vi "900x 9870 Interrupt Read (Sub).vi"(8 "error in":errorcluster, 9 "Number of bytes":i32, 11 "FPGA In":T1) -> (0 "error out":errorcluster, 1 "Byte Count":u32, 2 "Read Bytes":string, 3 "FPGA Out":T1, 4 "Timed Out":bool, 6 "FPGA Error":errorcluster)   [LabVIEW 2012]
uses:
  900x INT FPGA Reference.ctl
  FPGA Function.ctl
  <vilib>/Utility/error.llb/Error Cluster From Error Code.vi
  <vilib>/rvi/errors/niLvFpgaAdjustHostInterfaceError.vi
  <vilib>/rvi/interface/nirviReadWriteControl/nirviReadWriteControl.xnode
  FPGA Bitfiles/NI-987xSerialLoo_FPGATarget3_9870InterfaceInt_BB93BC1A.lvbitx
  Program Files (x86)/National Instruments/LabVIEW 2012/examples/CompactRIO/Module Specific/NI 987x/Serial Loopback/VIs/9870 Interface Interrupt (FPGA).vi
  <vilib>/rvi/interface/nirviMethod/nirviMethod.xnode
  NiFpgaLv.dll
  <vilib>/FPGAPlugInAG/cRIO-9101/niLvFpga_AcknowledgeIrq_cRIO-9101.vi
  <vilib>/rvi/interface/nirviMethod/StockFPGA_InlinedMethodWaitForSingleIRQ.vi
  <vilib>/FPGAPlugInAG/cRIO-9101/niLvFpga_WaitOnIrq_cRIO-9101.vi
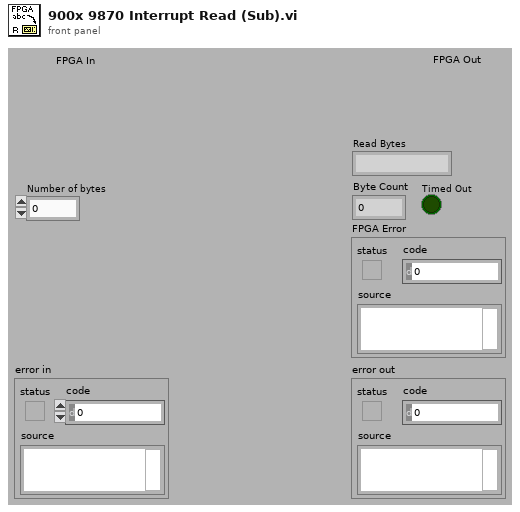
[diagram p1: front panel]
types:
  T1 = typedef "900x INT FPGA Reference.ctl" = refnum<k20>
  T2 = typedef "FPGA Function.ctl" = enum16{"Do Nothing", "Write", "Read"}
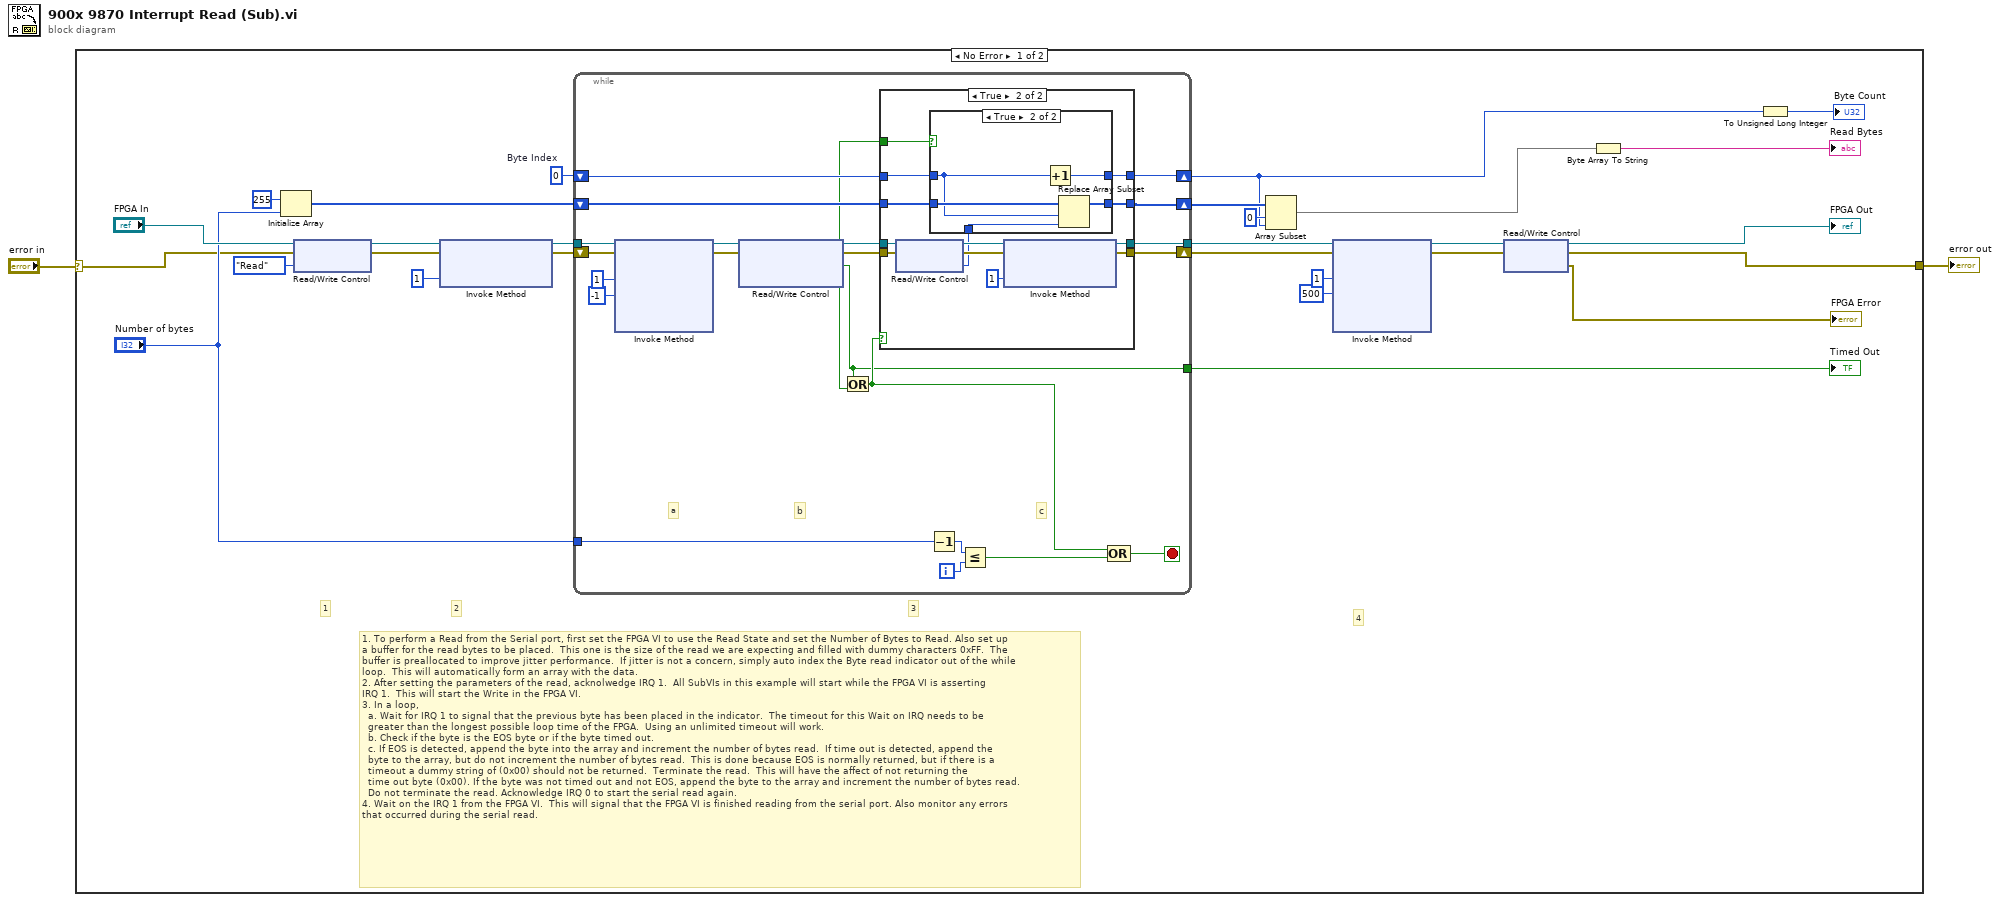
[diagram p0: block diagram]
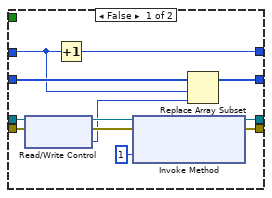
[diagram p2: hidden frame]
diagram:
  n1 = case shown="No Error" "error in" {
    selector: "error in" -> [w5 w85]
    tunnel: [w7 w85] -> w2
    frame No Error {
      w21 = 0  # Byte Index
      # "4"
      # "3"
      # "2"
      # "1"
      # "1. To perform a Read from the Serial port, first set the FPGA VI to use the Read State and set the Number of Bytes to Read. Also set up\na buffer for the read bytes to be placed.  This one is the size of the read we are expecting and filled with dummy characters 0xFF.  The\nbuffer is preallocated to improve jitter performance.  If jitter is not a concern, simply auto index the Byte read indicator out of the while\nloop.  This will automatically form an array with the data.\n2. After setting the parameters of the read, acknolwedge IRQ 1.  All SubVIs in this example will start while the FPGA VI is asserting \nIRQ 1.  This will start the Write in the FPGA VI.\n3. In a loop, \n  a. Wait for IRQ 1 to signal that the previous byte has been placed in the indicator.  The timeout for this Wait on IRQ needs to be\n  greater than the longest possible loop time of the FPGA.  Using an unlimited timeout will work.\n  b. Check if the byte is the EOS byte or if the byte timed out.\n  c. If EOS is detected, append the byte into the array and increment the number of bytes read.  If time out is detected, append the\n  byte to the array, but do not increment the number of bytes read.  This is done because EOS is normally returned, but if there is a \n  timeout a dummy string of (0x00) should not be returned.  Terminate the read.  This will have the affect of not returning the \n  time out byte (0x00). If the byte was not timed out and not EOS, append the byte to the array and increment the number of bytes read.  \n  Do not terminate the read. Acknowledge IRQ 0 to start the serial read again.\n4. Wait on the IRQ 1 from the FPGA VI.  This will signal that the FPGA VI is finished reading from the serial port. Also monitor any errors\nthat occurred during the serial read."
      n2 = Initialize Array(u8 255 ("element"), "Number of bytes") -> (w15:u8[])
      n3 = xnode "Read/Write Control"("FPGA VI Reference In"="FPGA In", "error in"=w5, "Op Control"=FPGA_Function."Read") -> ("FPGA VI Reference Out"=w29:T1, "error out"=w23:errorcluster)
      n4 = xnode "Invoke Method"("FPGA VI Reference In"=w29, "error in"=w23, "IRQ Number(s)"=1) -> ("FPGA VI Reference Out"=w28:T1, "error out"=w27:errorcluster)
      n5 = while {
        tunnel: [w52] -> w22
        shift-right: [w51] -> w24
        shift-left: w27 -> [w50]
        tunnel: w28 -> [w48]
        shift-right: [w46] -> w3
        shift-left: w21 -> [w47]
        tunnel: "Number of bytes" -> [w39]
        tunnel: [w32] -> w11
        shift-right: [w35] -> w14
        shift-left: w15 -> [w36]
        i -> [w40]
        stop <- w37 stop-if-true
        # "c"
        # "b"
        # "a"
        n6 = xnode "Invoke Method"("FPGA VI Reference In"=w48, "error in"=w50, "IRQ Number(s)"=1, "Timeout (ms)"=-1) -> ("FPGA VI Reference Out"=w45:T1, "error out"=w42:errorcluster)  [unwired: 2 out]
        n7 = xnode "Read/Write Control"("FPGA VI Reference In"=w45, "error in"=w42) -> ("FPGA VI Reference Out"=w44:T1, "error out"=w43:errorcluster, "Timed Out Read"=w32:bool, "EOS?"=w34:bool)
        n8 = Or(x=w32, y=w34) -> (x .or. y?=w33:bool)
        n9 = case shown="True" w33 {
          tunnel: [w64 w77] -> w52
          tunnel: [w63 w76] -> w51
          tunnel: w44 -> [w59 w72]
          tunnel: w43 -> [w58 w71]
          tunnel: w47 -> [w53 w66]
          tunnel: [w57 w67] -> w46
          tunnel: w36 -> [w55 w69]
          tunnel: [w56 w70] -> w35
          tunnel: w34 -> [_ w65]
          frame False {
            n10 = xnode "Read/Write Control"("FPGA VI Reference In"=w59, "error in"=w58) -> ("FPGA VI Reference Out"=w60:T1, "error out"=w61:errorcluster, "Byte read"=w54:u8)
            n11 = Increment(x=w53) -> (x+1=w57:i32)
            n12 = xnode "Invoke Method"("FPGA VI Reference In"=w60, "error in"=w61, "IRQ Number(s)"=1) -> ("FPGA VI Reference Out"=w64:T1, "error out"=w63:errorcluster)
            n13 = Replace Array Subset(array=w55, new element=w54, index=w53) -> (w56:u8[])
          }
          frame True {
            n14 = xnode "Read/Write Control"("FPGA VI Reference In"=w72, "error in"=w71) -> ("FPGA VI Reference Out"=w73:T1, "error out"=w74:errorcluster, "Byte read"=w68:u8)
            n15 = case shown="True" w65 {
              tunnel: [w79 w84] -> w70
              tunnel: w69 -> [w79 w83]
              tunnel: w68 -> [_ w82]
              tunnel: [w78 w80] -> w67
              tunnel: w66 -> [w78 w81]
              frame False {
              }
              frame True {
                n16 = Increment(x=w81) -> (x+1=w80:i32)
                n17 = Replace Array Subset(array=w83, new element=w82, index=w81) -> (w84:u8[])
              }
            }
            n18 = xnode "Invoke Method"("FPGA VI Reference In"=w73, "error in"=w74, "IRQ Number(s)"=1) -> ("FPGA VI Reference Out"=w77:T1, "error out"=w76:errorcluster)
          }
        }
        n19 = Decrement(x=w39) -> (x-1=w38:i32)
        n20 = Less Or Equal?(x=w38, y=w40) -> (x <= y?=w41:bool)
        n21 = Compound Arithmetic op=OR(w33, w41) -> (w37:bool)
      }
      "Timed Out" <- w11
      n22 = Array Subset(array=w14, index=0, length=w3) -> (w12:u8[])
      n23 = xnode "Invoke Method"("FPGA VI Reference In"=w22, "error in"=w24, "IRQ Number(s)"=1, "Timeout (ms)"=500) -> ("FPGA VI Reference Out"=w10:T1, "error out"=w9:errorcluster)  [unwired: 2 out]
      n24 = xnode "Read/Write Control"("FPGA VI Reference In"=w10, "error in"=w9) -> ("FPGA VI Reference Out"=→"FPGA Out":T1, "error out"=w7:errorcluster, "error out"=→"FPGA Error":errorcluster)
      n25 = Byte Array To String(unsigned byte array=w12) -> (string=→"Read Bytes":string)
      n26 = To Unsigned Long Integer(number=w3) -> (unsigned 32bit integer=→"Byte Count":u32)
    }
    frame Error {
    }
  }
  "error out" <- w2
